vi "TimeInfoCLOSE_old.vi"(7 "error in (no error)":errorcluster, 9 "Minor Time":u32, 10 "Major Time":u32) -> (1 "Close":cluster{"Time":string, "Error":string})   [LabVIEW 2015]
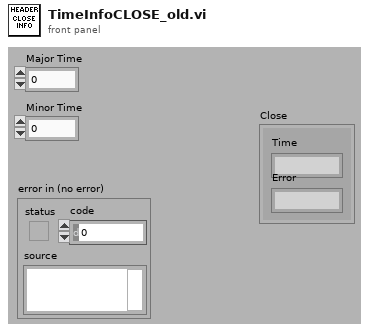
[diagram p1: front panel]
types:
  T1 = cluster{"  Close Time":string, "Close Error":string}
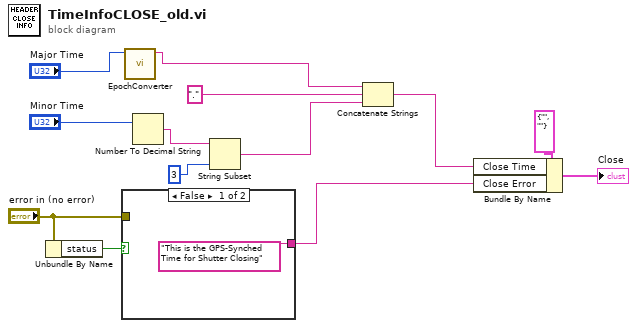
[diagram p0: block diagram]
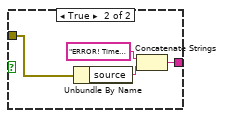
[diagram p2: hidden frame]
diagram:
  n1 = Unbundle By Name("error in (no error)") -> ("status"=w11:bool)
  n2 = case shown="False" w11 {
    tunnel: "error in (no error)" -> [_ w18]
    tunnel: ["This is the GPS-Synched Time for Shutter Closing" w15] -> w7
    frame False {
    }
    frame True {
      n3 = Unbundle By Name(w18) -> ("source"=w16:string)
      n4 = Concatenate Strings("ERROR! Time may be Invalid.  Source: ", w16) -> (w15:string)
    }
  }
  n5 = call "EpochConverter.vi"("Epoch time"="Major Time") -> ("String"=w4:string)  [unwired: 9 in, 1 out]
  n6 = Number To Decimal String(number="Minor Time") -> (decimal integer string=w3:string)  [unwired: 1 in]
  n7 = String Subset(string=w3, length (rest)=3) -> (substring=w2:string)  [unwired: 1 in]
  n8 = Concatenate Strings(w4, ".", w2) -> (w8:string)
  n9 = Bundle By Name(cluster=T1 {"  Close Time"="", "Close Error"=""}, "Close Time"=w8, "Close Error"=w7) -> (→"Close":T1)
